vi "Parse-Wall_Tunneling.vi"(6 "Tunnal All (F)":bool, 10 "Walls to Tunnel":i32=2, 11 "Line to Parse":u32[](array[numeric]) format="%06x") -> (1 "Tile Type":T2[](array[typedef]), 2 "Wall Data":T1[](array[typedef]), 3 "Wall Center Index":i32[](array[numeric]), 4 "Wall Thickness (px)":i32)   [LabVIEW 2020]
doc: "<B>Description:</B> Tunnels through the specified number of walls. Retuns the the index where the wall ends. \n\n<B>Date:</B> 04/2019\n<B>Author:</B> Luke Jarocki, Choose Movement Consulting, LLC"
uses:
  Controls/TileColor.ctl
  Controls/Wall Data.ctl
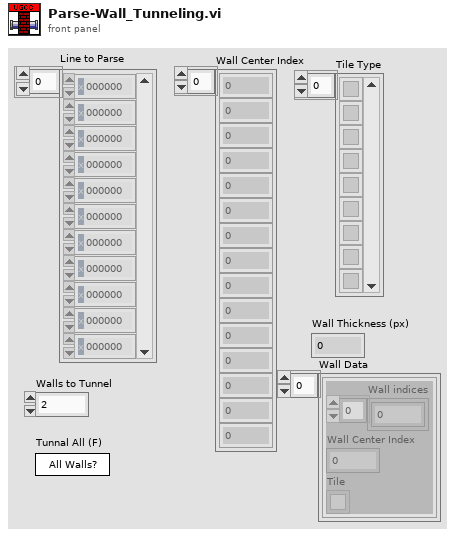
[diagram p1: front panel]
types:
  T1 = typedef "Wall Data.ctl" = cluster{"Wall indices":i32[], "Wall Center Index":i32, "Tile":T2}
  T2 = typedef "TileColor.ctl" = u16
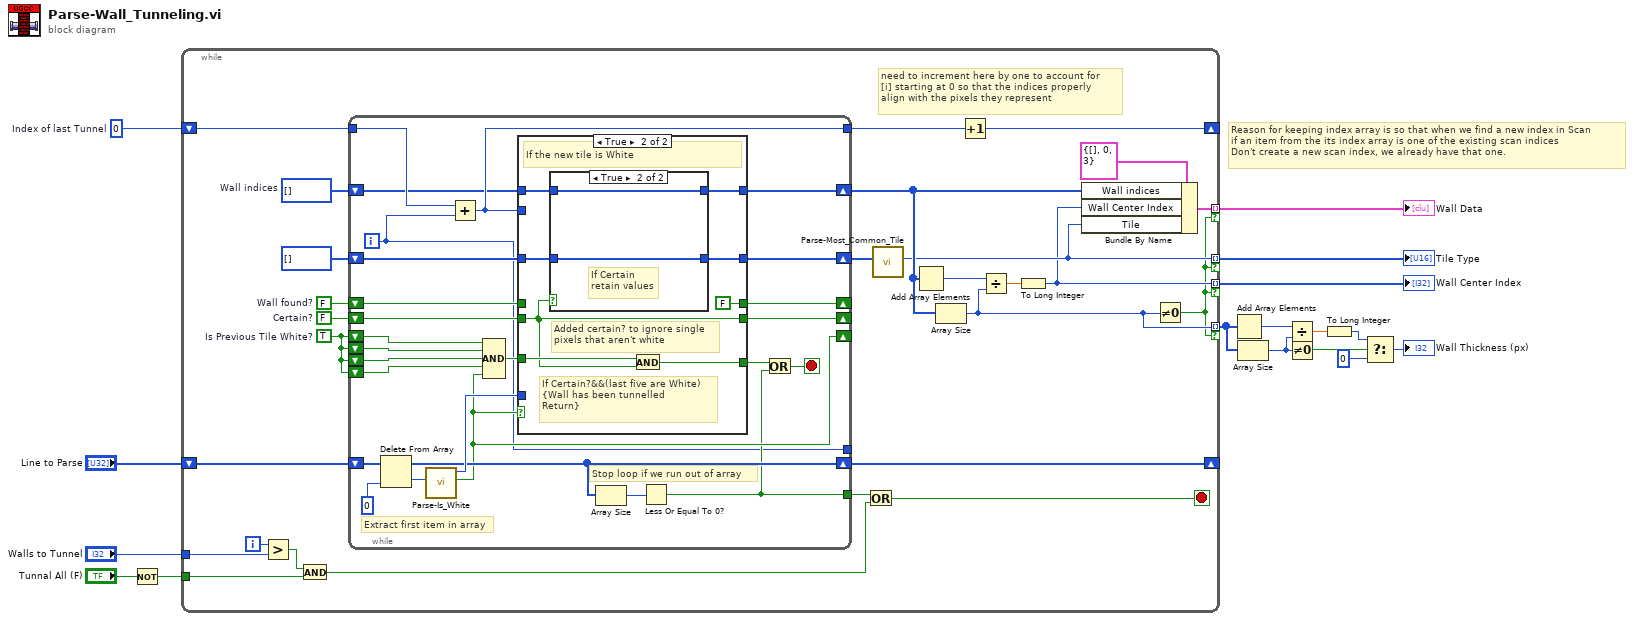
[diagram p0: block diagram]
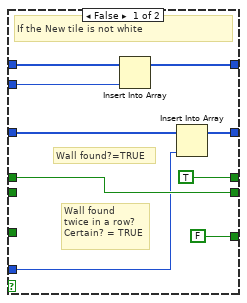
[diagram p2: hidden frame]
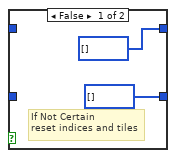
[diagram p3: hidden frame]
diagram:
  w15 = 0  # Index of last Tunnel
  # "Reason for keeping index array is so that when we find a new index in Scan\nif an item from the its index array is one of the existing scan indices\nDon't create a new scan index, we already have that one."
  n1 = Not(x="Tunnal All (F)") -> (.not. x?=w12:bool)
  n2 = while {
    tunnel: "Walls to Tunnel" -> [w42]
    shift-right: [w36] -> _
    shift-left: "Line to Parse" -> [w43]
    shift-right: [w17] -> _
    shift-left: w15 -> [w40]
    tunnel: [w21] -> w6 mode=indexing if=w18
    tunnel: w12 -> [w29]
    tunnel: [w25] -> w11 mode=indexing if=w18
    tunnel: [w20] -> w8 mode=indexing if=w18
    tunnel: [w19] -> w7 mode=indexing if=w18
    i -> [w35]
    stop <- w31 stop-if-true
    w34 = FALSE  # Certain?
    w37 = i32[] []  # Wall indices
    w41 = FALSE  # Wall found?
    w38 = TRUE  # Is Previous Tile White?
    # "need to increment here by one to account for\n[i] starting at 0 so that the indices properly\nalign with the pixels they represent"
    n3 = Greater?(x=w35, y=w42) -> (0:w30:bool)
    n4 = And(x=w30, y=w29) -> (x .and. y?=w28:bool)
    n5 = while {
      shift-right: [w50] -> w36
      shift-left: w43 -> [w69]
      shift-right: [w48] -> _
      shift-left: w38 -> [w60]
      shift-left: w38 -> [w64]
      shift-left: w38 -> [w65]
      shift-left: w38 -> [w66]
      shift-right: [w62] -> _
      shift-left: w41 -> [w61]
      tunnel: w40 -> [w58]
      tunnel: [w57] -> w39
      shift-right: [w55] -> w22
      shift-left: w37 -> [w56]
      shift-right: [w53] -> w32
      shift-left: T2[] [] -> [w54]
      shift-right: [w46] -> _
      shift-left: w34 -> [w47]
      tunnel: [w45] -> w27
      tunnel: [w44] -> _
      i -> [w44]
      stop <- w49 stop-if-true
      # "Stop loop if we run out of array"
      # "Extract first item in array"
      n6 = Delete From Array(array=w69, index=0) -> (deleted portion=w67:u32, array with subset deleted=w50:u32[])  [unwired: 1 in]
      n7 = call "Parse-Is_White.vi"("Color"=w67) -> ("Is White"=w48:bool, "Tile Color"=w63:T2)  [unwired: 8 in, 1 out]
      n8 = Add(x=w58, y=w44) -> (x+y=w57:i32)
      n9 = Compound Arithmetic op=AND(w60, w64, w65, w66, w48) -> (w59:bool)
      n10 = case shown="True" w48 {
        tunnel: w63 -> [w70 _]
        tunnel: [TRUE FALSE] -> w62
        tunnel: w61 -> [w73 _]
        tunnel: [FALSE w85] -> w51
        tunnel: w59 -> [_ w86]
        tunnel: w57 -> [w75 _]
        tunnel: w56 -> [w76 w81]
        tunnel: [w74 w82] -> w55
        tunnel: w54 -> [w72 w79]
        tunnel: [w71 w80] -> w53
        tunnel: w47 -> [_ w83]
        tunnel: [w73 w83] -> w46
        frame False {
          # "Wall found\ntwice in a row?\nCertain? = TRUE"
          # "Wall found?=TRUE"
          # "If the New tile is not white"
          n11 = Insert Into Array(array=w76, new element=w75) -> (w74:i32[])  [unwired: 1 in]
          n12 = Insert Into Array(array=w72, new element=w70) -> (w71:T2[])  [unwired: 1 in]
        }
        frame True {
          # "If Certain?&&(last five are White)\n{Wall has been tunnelled\nReturn}"
          # "Added certain? to ignore single\npixels that aren't white"
          # "If the new tile is White"
          n13 = case shown="True" w83 {
            tunnel: [i32[] [] w90] -> w82
            tunnel: w81 -> [_ w90]
            tunnel: [T2[] [] w89] -> w80
            tunnel: w79 -> [_ w89]
            frame False {
              # "If Not Certain\nreset indices and tiles"
            }
            frame True {
              # "If Certain\nretain values"
            }
          }
          n14 = And(x=w86, y=w83) -> (x .and. y?=w85:bool)
        }
      }
      n15 = Array Size(array=w50) -> (size(s)=w52:i32)
      n16 = Less Or Equal To 0?(x=w52) -> (x <= 0?=w45:bool)
      n17 = Or(x=w51, y=w45) -> (x .or. y?=w49:bool)
    }
    n18 = Or(x=w27, y=w28) -> (x .or. y?=w31:bool)
    n19 = call "Parse-Most_Common_Tile.vi"("Array"=w32) -> ("Tile"=w20:T2)  [unwired: 10 in]
    n20 = Add Array Elements(numeric array=w22) -> (sum=w26:i32)
    n21 = Array Size(array=w22) -> (size(s)=w25:i32)
    n22 = Increment(x=w39) -> (x+1=w17:i32)
    n23 = Divide(x=w26, y=w25) -> (x/y=w24:dbl)
    n24 = To Long Integer(number=w24) -> (32bit integer=w19:i32)
    n25 = Bundle By Name(cluster=T1 {"Wall indices"=[], "Wall Center Index"=0, "Tile"=3}, "Wall indices"=w22, "Wall Center Index"=w19, "Tile"=w20) -> (w21:T1)
    n26 = Not Equal To 0?(x=w25) -> (x != 0?=w18:bool)
  }
  "Wall Center Index" <- w7
  "Tile Type" <- w8
  "Wall Data" <- w6
  n27 = Add Array Elements(numeric array=w11) -> (sum=w10:i32)
  n28 = Array Size(array=w11) -> (size(s)=w5:i32)
  n29 = Divide(x=w10, y=w5) -> (x/y=w9:dbl)
  n30 = Not Equal To 0?(x=w5) -> (x != 0?=w4:bool)
  n31 = To Long Integer(number=w9) -> (32bit integer=w3:i32)
  n32 = Select(t=w3, s=w4, f=0) -> (s? t:f=→"Wall Thickness (px)":i32)
